vi "Apply Hardware Configurations.vi"(8 "error in (no error)":errorcluster, 9 "HW Config Object":refnum<class "HW Configuration.lvclass">, 10 "Device Name":string, 11 "Controller in":refnum<class "Controller.lvclass">) -> (0 "error out":errorcluster, 3 "Controller out":refnum<class "Controller.lvclass">)   [LabVIEW 2026, in "Controller Actor.lvlib" / "Controller.lvclass"]
uses:
  Controller.lvclass
  Hardware/HW Config/HW Configuration.lvclass
  Hardware/Hardware.lvclass
  Hardware/Hardware.lvclass/Hardware.ctl
  Controller.lvclass/Controller.ctl
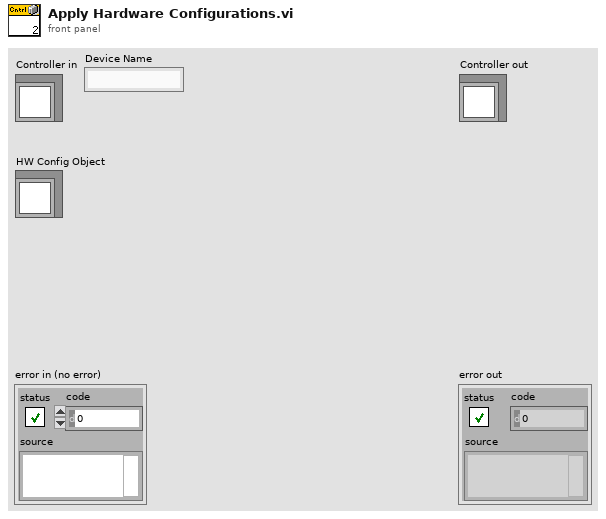
[diagram p1: front panel]
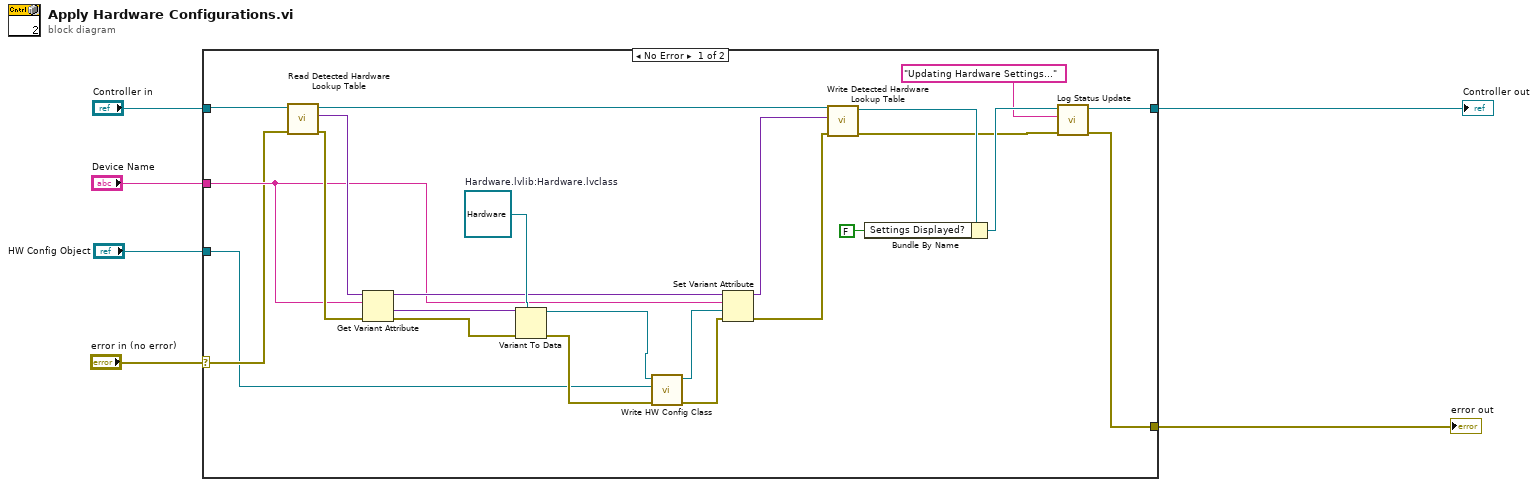
[diagram p0: block diagram]
diagram:
  n1 = case shown="No Error" "error in (no error)" {
    selector: "error in (no error)" -> [w17 w32]
    tunnel: [w13 w32] -> w5
    tunnel: [w15 w31] -> w3
    tunnel: "Controller in" -> [w20 w31]
    tunnel: "HW Config Object" -> [w9 _]
    tunnel: "Device Name" -> [w18 _]
    frame No Error {
      w27 = refnum<class "Hardware.lvclass"> refnum  # Hardware.lvlib:Hardware.lvclass
      n2 = call "Read Detected Hardware Lookup Table.vi"("error in (no error)"=w17, "Controller in"=w20) -> ("error out"=w29:errorcluster, "Detected Hardware Lookup Table"=w30:variant, "Controller out"=w19:refnum<class "Controller.lvclass">)  [unwired: 7 in]
      n3 = Get Variant Attribute(Variant=w30, name=w18, error in=w29) -> (duplicate Variant=w25:variant, value=w28:variant, error out=w26:errorcluster)  [unwired: 1 in, 1 out]
      n4 = Variant To Data(error in=w26, type=w27, Variant=w28) -> (data=w8:refnum<class "Hardware.lvclass">, error out=w11:errorcluster)
      n5 = call "Write HW Config Class.vi"("error in (no error)"=w11, "Hardware.lvlib:HW Configuration.lvclass"=w9, "Hardware in"=w8) -> ("error out"=w10:errorcluster, "Hardware out"=w7:refnum<class "Hardware.lvclass">)  [unwired: 7 in]
      n6 = Set Variant Attribute(Variant=w25, name=w18, value=w7, error in=w10) -> (Variant out=w24:variant, error out=w21:errorcluster)  [unwired: 1 out]
      n7 = call "Write Detected Hardware Lookup Table.vi"("error in (no error)"=w21, "Detected Hardware Lookup Table"=w24, "Controller in"=w19) -> ("error out"=w14:errorcluster, "Controller out"=w23:refnum<class "Controller.lvclass">)  [unwired: 7 in]
      n8 = Bundle By Name(cluster=w23, "Settings Displayed?"=FALSE) -> (w16:refnum<class "Controller.lvclass">)
      n9 = call-dynamic "Log Status Update.vi"("error in (no error)"=w14, "String"="Updating Hardware Settings...", "Controller in"=w16) -> ("error out"=w13:errorcluster, "Controller out"=w15:refnum<class "Controller.lvclass">)  [unwired: 7 in]
    }
    frame Error {
    }
  }
  "error out" <- w5
  "Controller out" <- w3
